vi "getPropertyType.vi"(8 "error in (no error)":errorcluster, 11 "IProperty in":refnum<class "IProperty.lvclass">) -> (0 "error out":errorcluster, 2 "Property Type out":T1 items=["Bool"=0, "Int"=1, "Float"=2, "String"=3, "List"=4, "Dict"=5, "Ratio"=6, "Procedure"=7, "Object"=8, "Function"=10, "Struct"=12, "Enumeration"=13, "Reference"=4096, "IndexSelection"=4097, "TypeSelection"=4098, "SparseSelection"=4099, "Undefined"=65535], 3 "IProperty out":refnum<class "IProperty.lvclass">)   [LabVIEW 2022 SP3, in "openDAQ.lvlib" / "IBaseObject.lvlib" / "IProperty.lvlib" / "IProperty.lvclass"]
uses:
  <instrlib>/openDAQ/Public/Classes/IProperty/IProperty.lvclass
  C:/Program Files (x86)/National Instruments/LabVIEW 2022/instr.lib/openDAQ/Public/Classes/IBaseObject/IBaseObject.lvclass
  <instrlib>/openDAQ/Public/Classes/IBaseObject/IBaseObject.lvclass/IBaseObject.ctl
  <instrlib>/openDAQ/Public/Classes/IBaseObject/Accessor/Read reference.vi
  <instrlib>/openDAQ/Public/Classes/IProperty/IProperty.lvclass/IProperty.ctl
  <instrlib>/openDAQ/Binaries/Windows/x86/copendaq32.dll
  <instrlib>/openDAQ/Public/TypeDef/PropertyType.ctl
  <instrlib>/openDAQ/openDAQ.lvlib
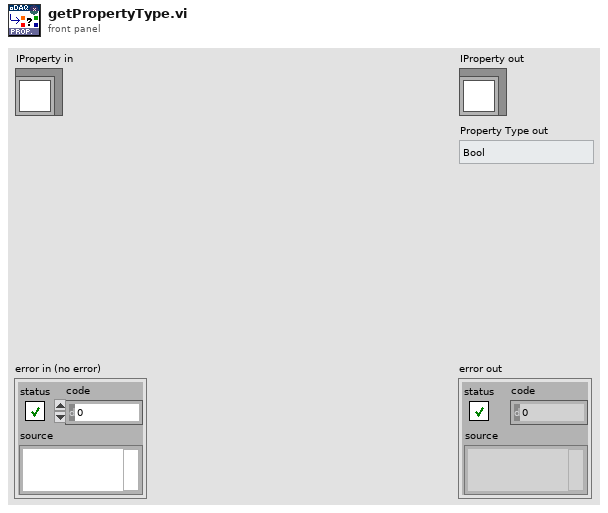
[diagram p1: front panel]
types:
  T1 = typedef "openDAQ.lvlib/PropertyType.ctl" = u16
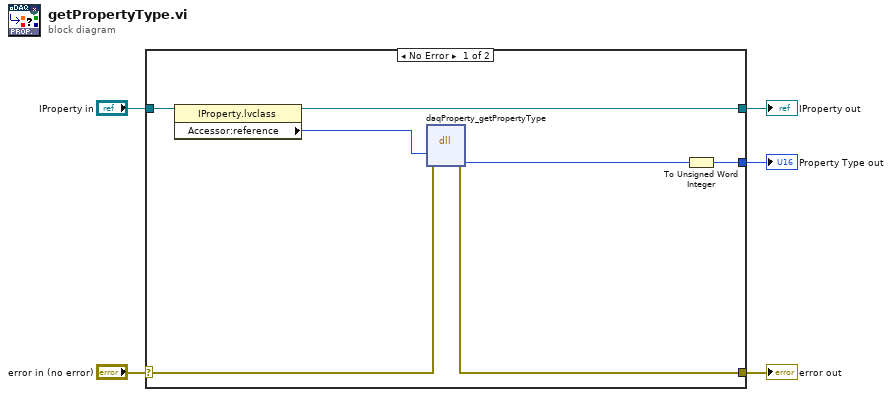
[diagram p0: block diagram]
diagram:
  n1 = case shown="No Error" "error in (no error)" {
    selector: "error in (no error)" -> [w11 w14]
    tunnel: [w10 w14] -> w4
    tunnel: [w9 w13] -> w2
    tunnel: "IProperty in" -> [w12 w13]
    tunnel: [w6 _] -> w1
    frame No Error {
      n2 = property class="IProperty.lvclass"(reference=w12) -> (reference out=w9:refnum<class "IProperty.lvclass">, "Accessor:reference"=w8:i64)  [unwired: 1 in, 1 out]
      n3 = dll-call lib="C:/Program Files (x86)/National Instruments/LabVIEW 2022/instr.lib/openDAQ/Binaries/Windows/x86/copendaq*.*" fn="daqProperty_getPropertyType"(error in=w11, "property"=w8) -> (error out=w10:errorcluster, "type"=w7:i64)  [unwired: 5 in, 1 out]
      n4 = To Unsigned Word Integer(number=w7) -> (unsigned 16bit integer=w6:u16)
    }
    frame Error {
    }
  }
  "error out" <- w4
  "IProperty out" <- w2
  "Property Type out" <- w1
